vi "Read PID.vi"(8 "error in (no error)":errorcluster, 11 "ThermPID in":refnum<class "ThermPID.lvclass">) -> (0 "error out":errorcluster, 2 "register values":dbl[](array[numeric]), 3 "ThermPID out":refnum<class "ThermPID.lvclass">)   [LabVIEW 2023, in "ThermPID.lvclass"]
uses:
  ThermPID.lvclass
  ThermPID.lvclass/ThermPID.ctl
  PIDController/PIDController.lvclass
  PIDModBus/Controls/Register Enum.ctl
  PIDModBus/PIDModbus.lvlib
  <vilib>/NI/Modbus Library/API/Master/Modbus Master.lvclass
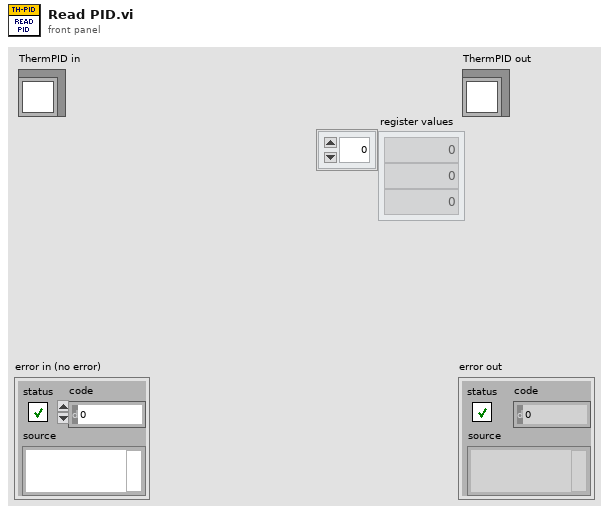
[diagram p1: front panel]
types:
  T1 = typedef "PIDModbus.lvlib/Register Enum.ctl" = u16
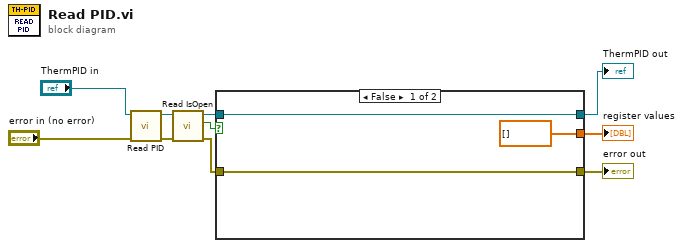
[diagram p0: block diagram]
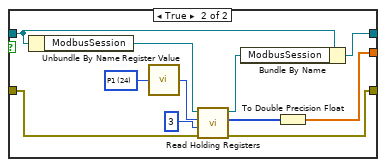
[diagram p2: hidden frame]
diagram:
  n1 = call-parent "Read PID.vi"("error in (no error)"="error in (no error)", "PIDController in"="ThermPID in") -> ("error out"=w3:errorcluster, "PIDController out"=w5:refnum<class "ThermPID.lvclass">)  [unwired: 8 in]
  n2 = call-dynamic "Read IsOpen.vi"("error in (no error)"=w3, "PIDController in"=w5) -> ("error out"=w2:errorcluster, "IsOpen"=w1:bool, "PIDController out"=w4:refnum<class "ThermPID.lvclass">)  [unwired: 7 in]
  n3 = case shown="False" w1 {
    tunnel: [dbl[] [] w20] -> w8
    tunnel: [w12 w18] -> w7
    tunnel: [w13 w17] -> w6
    tunnel: w4 -> [w13 w15]
    tunnel: w2 -> [w12 w14]
    frame False {
    }
    frame True {
      w22 = T1 24 items=["PV"=0, "SV"=5, "P1"=24, "I1"=25, "D1"=26] ("Register")
      n4 = Unbundle By Name(w15) -> ("ModbusSession"=w19:refnum<class "Modbus Master.lvclass">)
      n5 = call "Register Value.vi"("Register"=w22) -> ("RegAddr (Hex)"=w21:u16)
      n6 = call-dynamic "Read Holding Registers.vi"("error in"=w14, "number of inputs"=u16 3, "starting address"=w21, "Modbus master in"=w19) -> ("error out"=w18:errorcluster, "register values"=w24:u16[], "Modbus master out"=w16:refnum<class "Modbus Master.lvclass">)  [unwired: 5 in]
      n7 = Bundle By Name(cluster=w15, "ModbusSession"=w16) -> (w17:refnum<class "ThermPID.lvclass">)
      n8 = To Double Precision Float(number=w24) -> (double precision float=w20:dbl[])
    }
  }
  "error out" <- w7
  "ThermPID out" <- w6
  "register values" <- w8
